vi "RTS Update Owner Name.vi"(8 "Error In":errorcluster, 9 "Insert Value":string, 10 "Tree Selection":T1="Select Room/Stall", 11 "Station Owner Names Input":string[](array[string])) -> (0 "Error Out":errorcluster, 3 "Station Owner Names Output":string[](array[string]))   [LabVIEW 2016]
uses:
  Type Definitions/RTS Room Selector.ctl
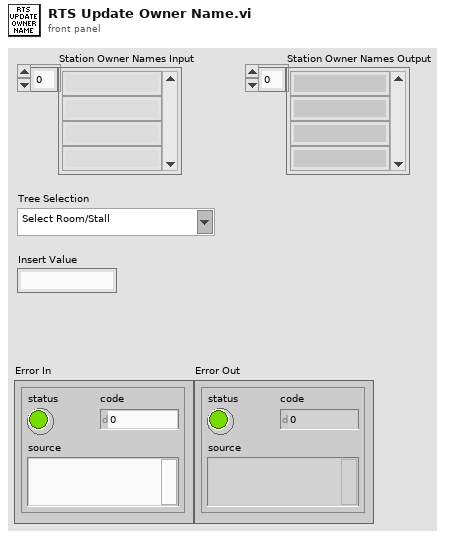
[diagram p1: front panel]
types:
  T1 = typedef "RTS Room Selector.ctl" = string
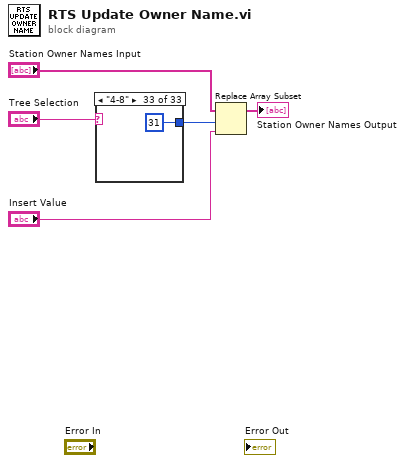
[diagram p0: block diagram]
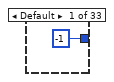
[diagram p2: hidden frame]
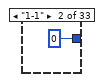
[diagram p3: hidden frame]
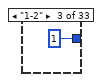
[diagram p4: hidden frame]
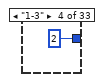
[diagram p5: hidden frame]
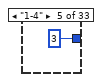
[diagram p6: hidden frame]
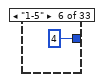
[diagram p7: hidden frame]
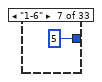
[diagram p8: hidden frame]
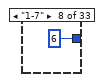
[diagram p9: hidden frame]
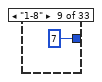
[diagram p10: hidden frame]
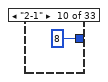
[diagram p11: hidden frame]
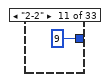
[diagram p12: hidden frame]
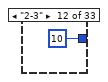
[diagram p13: hidden frame]
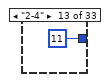
[diagram p14: hidden frame]
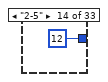
[diagram p15: hidden frame]
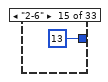
[diagram p16: hidden frame]
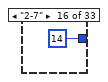
[diagram p17: hidden frame]
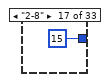
[diagram p18: hidden frame]
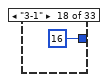
[diagram p19: hidden frame]
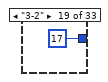
[diagram p20: hidden frame]
diagram:
  n1 = case shown="\"4-8\"" "Tree Selection" {
    tunnel: [-1 0 1 2 3 4 5 6 7 8 9 10 11 12 13 14 15 16 17 18 19 20 21 22 23 24 25 26 27 28 29 30 31] -> w3
    frame Default {
    }
    frame "1-1" {
    }
    frame "1-2" {
    }
    frame "1-3" {
    }
    frame "1-4" {
    }
    frame "1-5" {
    }
    frame "1-6" {
    }
    frame "1-7" {
    }
    frame "1-8" {
    }
    frame "2-1" {
    }
    frame "2-2" {
    }
    frame "2-3" {
    }
    frame "2-4" {
    }
    frame "2-5" {
    }
    frame "2-6" {
    }
    frame "2-7" {
    }
    frame "2-8" {
    }
    frame "3-1" {
    }
    frame "3-2" {
    }
    frame "3-3" {
    }
    frame "3-4" {
    }
    frame "3-5" {
    }
    frame "3-6" {
    }
    frame "3-7" {
    }
    frame "3-8" {
    }
    frame "4-1" {
    }
    frame "4-2" {
    }
    frame "4-3" {
    }
    frame "4-4" {
    }
    frame "4-5" {
    }
    frame "4-6" {
    }
    frame "4-7" {
    }
    frame "4-8" {
    }
  }
  n2 = Replace Array Subset(array="Station Owner Names Input", new element="Insert Value", index=w3) -> (→"Station Owner Names Output":string[])
